vi "build_reply.vi"() -> (2 "output array":u8[](array[numeric]))   [LabVIEW 2024]
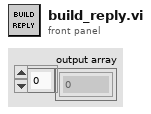
[diagram p1: front panel]
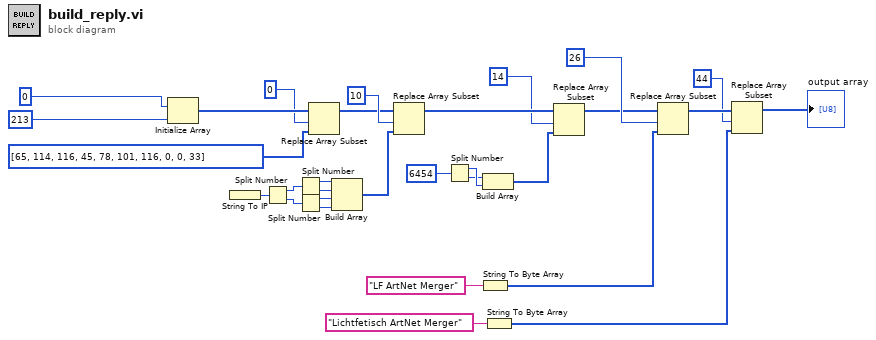
[diagram p0: block diagram]
diagram:
  n1 = Initialize Array(u8 0, 213 ("dimension size")) -> (w19:u8[])
  n2 = String To IP() -> (0:w30:u32)  [unwired: 1 in]
  n3 = Split Number(x=w30) -> (hi(x)=w29:u16, lo(x)=w28:u16)
  n4 = Split Number(x=w29) -> (hi(x)=w27:u8, lo(x)=w26:u8)
  n5 = Split Number(x=w28) -> (hi(x)=w25:u8, lo(x)=w24:u8)
  n6 = Replace Array Subset(array=w19, new element=u8[] [65, 114, 116, 45, 78, 101, 116, 0, 0, 33] ("Vorzeichenloses Byte-Array"), index=0) -> (w16:u8[])
  n7 = Build Array(w27, w26, w25, w24) -> (w20:u8[])
  n8 = Replace Array Subset(array=w16, new element=w20, index=10) -> (w12:u8[])
  n9 = Split Number(x=u16 6454) -> (hi(x)=w14:u8, lo(x)=w13:u8)
  n10 = String To Byte Array(string="LF ArtNet Merger") -> (unsigned byte array=w8:u8[])
  n11 = Build Array(w13, w14) -> (w10:u8[])
  n12 = String To Byte Array(string="Lichtfetisch ArtNet Merger") -> (unsigned byte array=w3:u8[])
  n13 = Replace Array Subset(array=w12, new element=w10, index=14) -> (w6:u8[])
  n14 = Replace Array Subset(array=w6, new element=w8, index=26) -> (w4:u8[])
  n15 = Replace Array Subset(array=w4, new element=w3, index=44) -> (→"output array":u8[])
